vi "GetDelay.vi"(8 "error in":errorcluster, 11 "Count":i32) -> (0 "error out":errorcluster, 3 "Delay":u32)   [LabVIEW 2012, in "Spinner.xctl"]
uses:
  Spinner.xctl
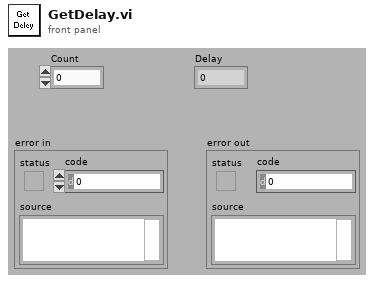
[diagram p1: front panel]
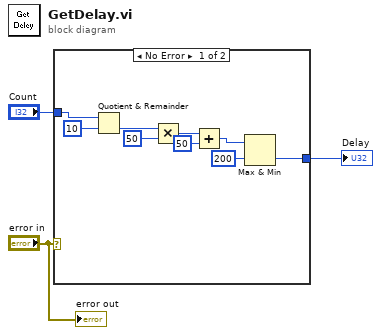
[diagram p0: block diagram]
diagram:
  n1 = case shown="No Error" "error in" {
    tunnel: "Count" -> [w12 _]
    tunnel: [w4 _] -> w2
    frame No Error {
      n2 = Quotient & Remainder(x=w12, y=10) -> (floor(x/y)=w10:i32)  [unwired: 1 out]
      n3 = Multiply(x=w10, y=50) -> (x*y=w9:i32)
      n4 = Add(x=w9, y=50) -> (x+y=w7:i32)
      n5 = Max & Min(x=w7, y=200) -> (min(x,y)=w4:i32)  [unwired: 1 out]
    }
    frame Error {
    }
  }
  "Delay" <- w2
  "error out" <- "error in"
